vi "entradaDeDados.vi"() -> ()   [LabVIEW 2012]
panel:
  in  "print?":bool caption="Print da\ncurva(s)"
  out "Temperatura":dbl format="%#_3g"
  in  "Help Button":bool
  in  "sair":bool
  in  "Irradiância":dbl caption="Irradiância(W/cm²)"
  in  "nCurvas":i64=1 caption="Nº de curvas" min=1
  in  "T.J":dbl caption="Tensão do joelho" step=0.1
  in  "p.a.j":dbl caption="Pontos antes do joelho"
  in  "nMedições":i16=1 caption="N° medições por ponto" min=1
  in  "area":dbl caption="Área da célula(cm²)"
  in  "Tipo":string caption="Tipo da célula"
  in  "Formato":u16(ring) items=[".txt", ".csv"]
  in  "p.d.j":dbl caption="Pontos depois do joelho"
  in  "T.M":dbl caption="Tensão máxima" step=0.1
  in  "Nome da célula":string
  in  "Local":path
  in  "Delay(ms)":dbl
  in  "Start":bool
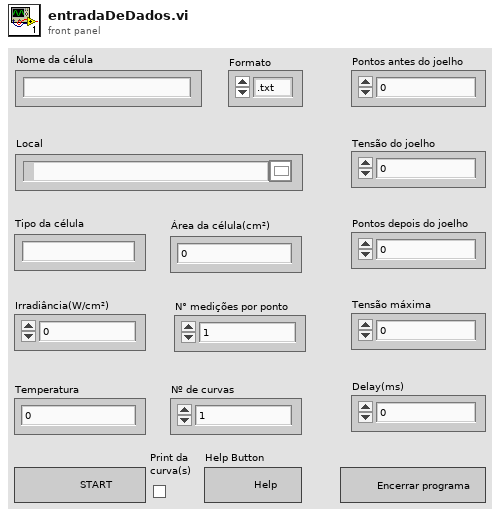
[diagram p1: front panel]
types:
  T1 = typedef "imagedata.ctl" = cluster{"image type":i32, "image depth":i32, "image":u8[], "mask":u8[], "colors":u32[], "Rectangle":cluster{"left":i16, "top":i16, "right":i16, "bottom":i16}}
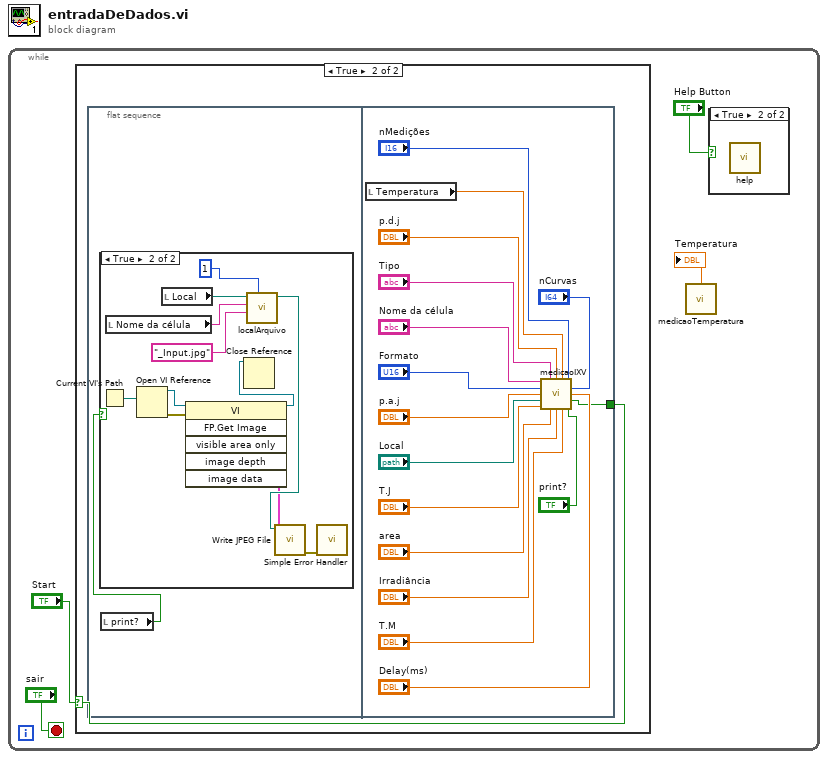
[diagram p0: block diagram]
diagram:
  n1 = while {
    stop <- "sair" stop-if-true
    n2 = case shown="True" "Start" {
      selector: "Start" -> [_ w5]
      frame False {
      }
      frame True {
        n3 = flat-sequence {
          tunnel: w5 -> [w18]
          frame #0 {
            n4 = local read "print?"() -> (w6:bool)
            n5 = case shown="True" w6 {
              frame False {
              }
              frame True {
                n6 = Current VI's Path() -> (path=w15:path)
                n7 = local read "Nome da célula"() -> (w11:string)
                n8 = Open VI Reference(vi path=w15) -> (vi reference=w16:refnum<vi>, error out=w17:errorcluster)  [unwired: 5 in]
                n9 = local read "Local"() -> (w12:path)
                n10 = invoke class="VI" method="FP.Get Image"(reference=w16, error in=w17) -> (reference out=w14:refnum<vi>, "image data"=w7:T1)  [unwired: 4 in, 4 out]
                n11 = Close Reference(reference=w14) -> ()  [unwired: 1 in, 1 out]
                n12 = call "localArquivo.vi"("quantidadeDeArquivos"=i16 1, "extensão"="_Input.jpg", "Nome do arquivo"=w11, "Local"=w12) -> ("Path"=w8:path)  [unwired: 7 in]
                n13 = call <vilib>:"Write JPEG File.vi"("image data"=w7, "path to JPEG file"=w8) -> ("error out"=w13:errorcluster)  [unwired: 8 in, 1 out]
                n14 = call <vilib>:"Simple Error Handler.vi"("error in (no error)"=w13) -> ()  [unwired: 4 in, 5 out]
              }
            }
          }
          frame #1 {
            n15 = local read "Temperatura"() -> (w32:dbl)
            n16 = call "medicaoIXV.vi"("Nome da célula"="Nome da célula", "Tipo"="Tipo", "p.d.j"="p.d.j", "temperatura"=w32, "nMedições"="nMedições", "Formato"="Formato", "nCurvas"="nCurvas", "p.a.j"="p.a.j", "Delay(ms)"="Delay(ms)", "Local"="Local", "Start"=w18, "T.J"="T.J", "area"="area", "Irradiância"="Irradiância", "T.M"="T.M", "print?"="print?") -> ()
          }
        }
      }
    }
    n17 = call "medicaoTemperatura.vi"() -> ("data"=→"Temperatura":dbl)  [unwired: 11 in]
    n18 = case shown="True" "Help Button" {
      frame False {
      }
      frame True {
        n19 = call "help.vi"() -> ()  [unwired: 11 in, 1 out]
      }
    }
  }
